vi "circular_mask.vi"(6 "CentreY":dbl=-1.0, 7 "Centre X":dbl=-1.0, 9 "Radius":dbl=-1.0, 10 "size":i32=256) -> (2 "Mask Array":i16[][](array[numeric]))   [LabVIEW 2016]
doc: "Creates a circular mask. Set centreX or centreY to -1 to centre mask. Set radius to -1 for circle to fill the array."
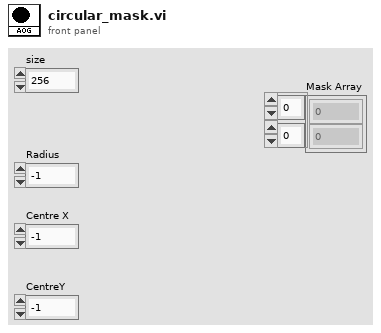
[diagram p1: front panel]
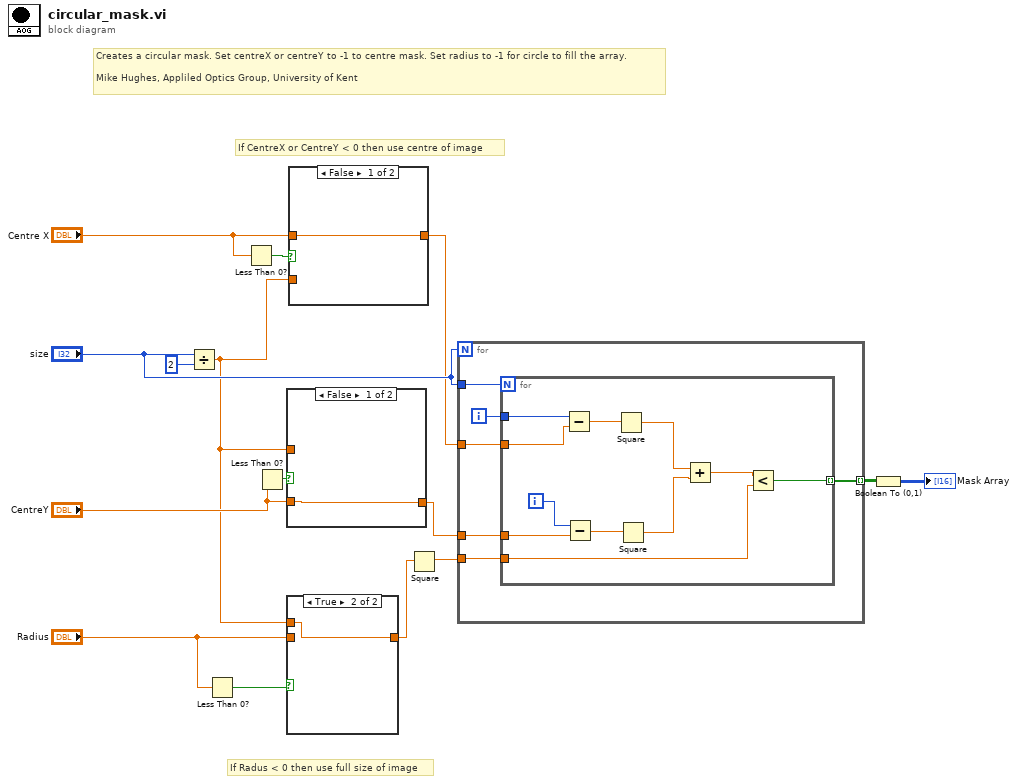
[diagram p0: block diagram]
diagram:
  # "Creates a circular mask. Set centreX or centreY to -1 to centre mask. Set radius to -1 for circle to fill the array.\n\nMike Hughes, Appliled Optics Group, University of Kent"
  # "If Radus < 0 then use full size of image"
  # "If CentreX or CentreY < 0 then use centre of image"
  n1 = Divide(x="size", y=2) -> (x/y=w1:dbl)
  n2 = Less Than 0?(x="Radius") -> (x < 0?=w4:bool)
  n3 = Less Than 0?(x="Centre X") -> (x < 0?=w9:bool)
  n4 = Less Than 0?(x="CentreY") -> (x < 0?=w7:bool)
  n5 = case shown="False" w7 {
    tunnel: "CentreY" -> [w16 _]
    tunnel: [w16 w17] -> w5
    tunnel: w1 -> [_ w17]
    frame False {
    }
    frame True {
    }
  }
  n6 = case shown="True" w4 {
    tunnel: "Radius" -> [w18 _]
    tunnel: [w18 w19] -> w2
    tunnel: w1 -> [_ w19]
    frame False {
    }
    frame True {
    }
  }
  n7 = case shown="False" w9 {
    tunnel: w1 -> [_ w21]
    tunnel: [w20 w21] -> w10
    tunnel: "Centre X" -> [w20 _]
    frame False {
    }
    frame True {
    }
  }
  n8 = Square(x=w2) -> (x^2=w15:dbl)
  n9 = for {
    N: "size" -> [_]
    tunnel: "size" -> [w27]
    tunnel: w10 -> [w25]
    tunnel: w15 -> [w24]
    tunnel: [w23] -> w14 mode=indexing
    tunnel: w5 -> [w22]
    i -> [w26]
    n10 = for {
      N: w27 -> [_]
      tunnel: w26 -> [w38]
      tunnel: w25 -> [w36]
      tunnel: w24 -> [w30]
      tunnel: [w29] -> w23 mode=indexing
      tunnel: w22 -> [w28]
      i -> [w37]
      n11 = Subtract(x=w38, y=w36) -> (x-y=w35:dbl)
      n12 = Subtract(x=w37, y=w28) -> (x-y=w34:dbl)
      n13 = Square(x=w35) -> (x^2=w32:dbl)
      n14 = Square(x=w34) -> (x^2=w33:dbl)
      n15 = Add(x=w32, y=w33) -> (x+y=w31:dbl)
      n16 = Less?(x=w31, y=w30) -> (x < y?=w29:bool)
    }
  }
  n17 = Boolean To (0,1)(Boolean=w14) -> (0, 1=→"Mask Array":i16[][])
